vi "FACTORY PATTERN.vi"() -> (3 "class":string[](array[string]))   [LabVIEW 2020]
uses:
  Libraries/FGen/Generador/Generador.lvclass
  Libraries/FGen/GeneradorAmplificado/GeneradorAmplificado.lvclass
  C:/Users/salma/IVSalma2P_2/Libraries/FGen/Generador/Generador.lvclass
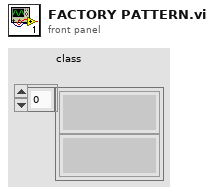
[diagram p1: front panel]
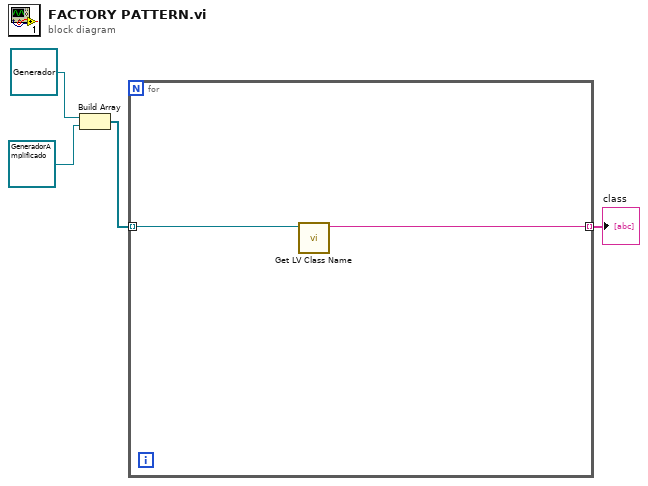
[diagram p0: block diagram]
diagram:
  n1 = Build Array(refnum<class "Generador.lvclass"> refnum ("FGen.lvlib:Generator"), refnum<class "GeneradorAmplificado.lvclass"> refnum ("FGen.lvlib:GeneradorAmplificado.lvclass")) -> (w2:refnum<class "Generador.lvclass">[])
  n2 = for {
    tunnel: w2 -> [w6] mode=indexing
    tunnel: [w5] -> w1 mode=indexing
    n3 = call <vilib>:"Get LV Class Name.vi"("object"=w6) -> ("class name"=w5:string)  [unwired: 9 in, 1 out]
  }
  "class" <- w1
